vi "IPFPCXT.vi"(3 "Number":cxt) -> (0 "Fractional part":cxt, 1 "Integer part":cxt)   [LabVIEW 2017, in "GPNumeric.lvlib"]
doc: "Splits floating point <B>Number</B> into <B>Integer part</B> and <B>Fractional part</B>.\n\nThis VI is inlined.\n\nSteen Schmidt\nGPower\n6/4 2014"
uses:
  GPNumeric.lvlib
panel:
  # "Copyright © 2014\nGPower\nSee enclosed license file for terms and conditions"
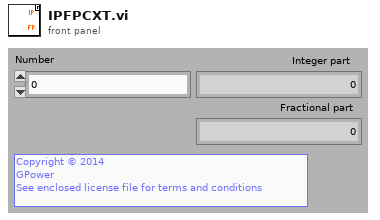
[diagram p1: front panel]
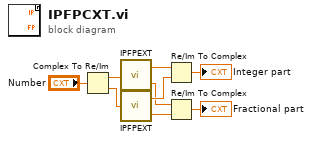
[diagram p0: block diagram]
diagram:
  n1 = Complex To Re/Im(x + iy="Number") -> (x=w8:ext, y=w7:ext)
  n2 = call "IPFPEXT.vi"("Number"=w8) -> ("Fractional part"=w3:ext, "Integer part"=w6:ext)  [unwired: 2 in]
  n3 = call "IPFPEXT.vi"("Number"=w7) -> ("Fractional part"=w2:ext, "Integer part"=w5:ext)  [unwired: 2 in]
  n4 = Re/Im To Complex(1:w5, 2:w6) -> (0:→"Integer part":cxt)
  n5 = Re/Im To Complex(1:w2, 2:w3) -> (0:→"Fractional part":cxt)
